vi "Routines.Compile.vi"(8 "error in (no error)":errorcluster, 11 "Section Ref in":T5 format="%.0x") -> (0 "error out":errorcluster, 1 "Routines":T1 {"Stop.Resp"."Signals"."Byte Order" items=["Little Endian", "Big Endian"]; "Stop.Resp"."Signals"."Data Type" items=["Signed", "Unsigned", "IEEE Float"]; "Stop.Cmd"."Signals"."Byte Order" items=["Little Endian", "Big Endian"]; "Stop.Cmd"."Signals"."Data Type" items=["Signed", "Unsigned", "IEEE Float"]; "Request.Resp"."Signals"."Byte Order" items=["Little Endian", "Big Endian"]; "Request.Resp"."Signals"."Data Type" items=["Signed", "Unsigned", "IEEE Float"]; "Request.Cmd"."Signals"."Byte Order" items=["Little Endian", "Big Endian"]; "Request.Cmd"."Signals"."Data Type" items=["Signed", "Unsigned", "IEEE Float"]; "Start.Resp"."Signals"."Byte Order" items=["Little Endian", "Big Endian"]; "Start.Resp"."Signals"."Data Type" items=["Signed", "Unsigned", "IEEE Float"]; "Start.Cmd"."Signals"."Byte Order" items=["Little Endian", "Big Endian"]; "Start.Cmd"."Signals"."Data Type" items=["Signed", "Unsigned", "IEEE Float"]}, 2 "Routines Refs":T6 {"Stop.Resp"."Signal Refs" format="%.0x"; "Stop.Cmd"."Signal Refs" format="%.0x"; "Request.Resp"."Signal Refs" format="%.0x"; "Request.Cmd"."Signal Refs" format="%.0x"; "Start.Resp"."Signal Refs" format="%.0x"; "Start.Cmd"."Signal Refs" format="%.0x"}, 3 "Section Ref out":T5 format="%.0x")   [LabVIEW 2015, in "Diagnostics Addon System Explorer.lvlib"]
uses:
  Diagnostics Addon System Explorer.lvlib
  <vilib>/NI Veristand/Custom Device API/Custom Device Item Ref.ctl
  Types/Routines.Refs.ctl
  Types/Frame.Ref.ctl
  Types/Routines.Compile.ctl
  Shared/Types/Frame.Compile.ctl
  Shared/Types/Type.ctl
  Shared/Types/Signal.ctl
  Types/FG.Action.ctl
  Signal.FG.vi
  <vilib>/NI Veristand/Custom Device API/NI VeriStand - Get Custom Device Channel Data.vi
  <vilib>/NI Veristand/Custom Device API/NI VeriStand - Get Item Description.vi
  <vilib>/NI Veristand/Custom Device API/NI VeriStand - Get Item Property.vi
  <vilib>/NI Veristand/Custom Device API/Get Item Property (String).vi
  <vilib>/NI Veristand/Custom Device API/Get Item Property (Double).vi
  <vilib>/NI Veristand/Custom Device API/Get Item Property (U32).vi
  <vilib>/NI/NI VeriStand Advanced SysDef API/SysDef API/SysDef.Property.Set.vi
  <vilib>/NI/NI VeriStand Advanced SysDef API/_SubVIs/SysDef.Property.Set.String.vi
  <vilib>/NI/NI VeriStand Advanced SysDef API/_SubVIs/SysDef.Property.Set.DBL.vi
  <vilib>/NI/NI VeriStand Advanced SysDef API/_SubVIs/SysDef.Property.Set.U32.vi
  Shared/SubVIs/Constants.vi
  <vilib>/NI Veristand/Custom Device Tools/Custom Device Utility Library/NI VeriStand - Search for Item by GUID.vi
  <vilib>/NI VeriStand/Custom Device Tools/Custom Device Utility Library/Custom Device Utility Library.lvlib
  <vilib>/NI VeriStand/Custom Device API/Custom Device API.lvlib
  Shared/Diagnostics Addon Shared.lvlib
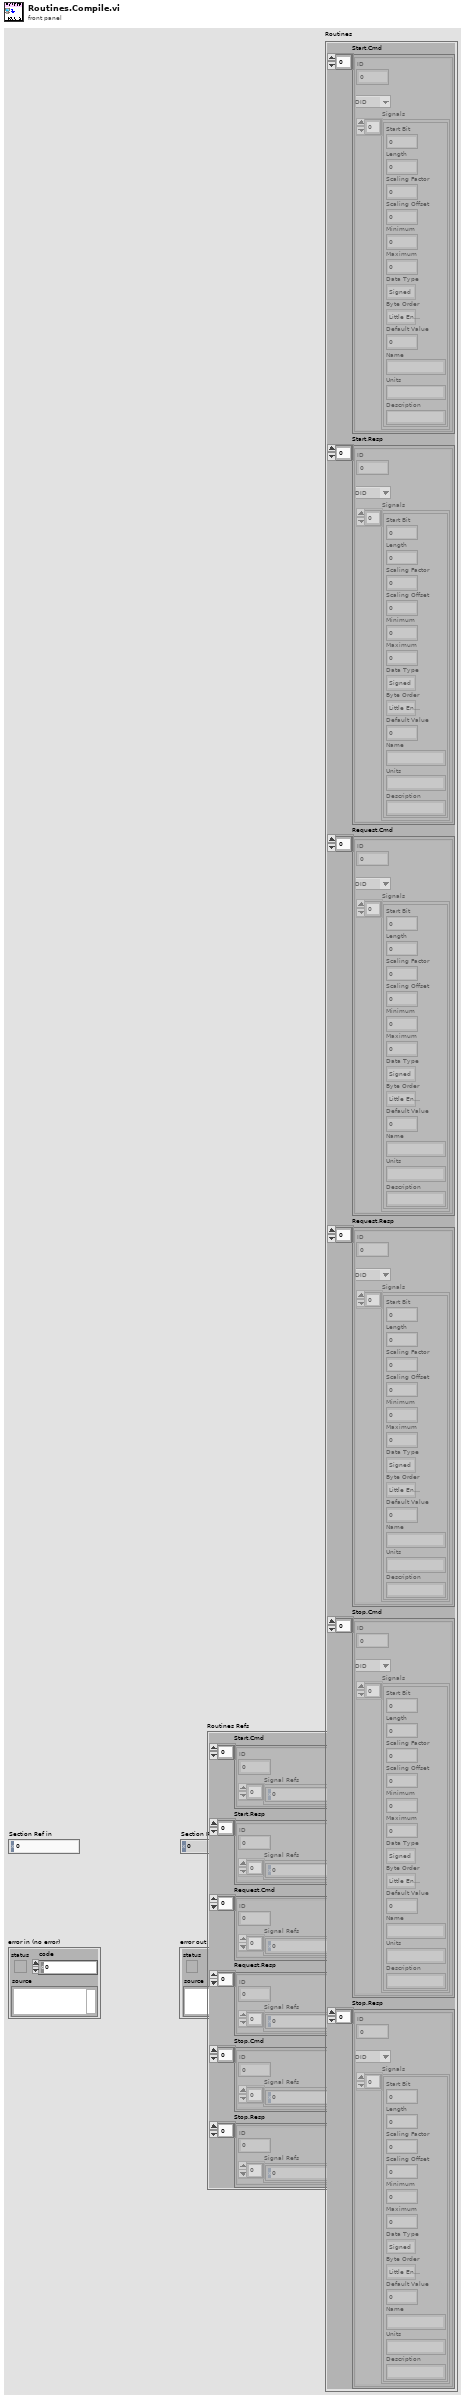
[diagram p1: front panel]
types:
  T1 = typedef "Diagnostics Addon System Explorer.lvlib/Routines.Compile.ctl" = cluster{"Start.Cmd":T2[], "Start.Resp":T2[], "Request.Cmd":T2[], "Request.Resp":T2[], "Stop.Cmd":T2[], "Stop.Resp":T2[]}
  T2 = typedef "Diagnostics Addon Shared.lvlib/Frame.Compile.ctl" = cluster{"ID":u32, "Type":T3, "Signals":T4[]}
  T3 = typedef "Diagnostics Addon Shared.lvlib/Type.ctl" = enum16{"DID", "CDID", "PID", "CPID", "Read Memory", "Write Memory", "DTC Control", "IO Cmd", "IO Resp", "Routine Start Cmd", "Routine Start Resp", "Routine Request Cmd", "Routine Request Resp", "Routine Stop Cmd", "Routine Stop Resp", "UserDefined Cmd", "UserDefined Rsp"}
  T4 = typedef "Diagnostics Addon Shared.lvlib/Signal.ctl" = cluster{"Start Bit":u32, "Length":u32, "Scaling Factor":dbl, "Scaling Offset":dbl, "Minimum":dbl, "Maximum":dbl, "Data Type":u32, "Byte Order":u32, "Default Value":dbl, "Name":string, "Units":string, "Description":string}
  T5 = typedef "Custom Device API.lvlib/Custom Device Item Ref.ctl" = u64
  T6 = typedef "Diagnostics Addon System Explorer.lvlib/Routines.Refs.ctl" = cluster{"Start.Cmd":T7[], "Start.Resp":T7[], "Request.Cmd":T7[], "Request.Resp":T7[], "Stop.Cmd":T7[], "Stop.Resp":T7[]}
  T7 = typedef "Diagnostics Addon System Explorer.lvlib/Frame.Ref.ctl" = cluster{"ID":u32, "Signal Refs":T5[]}
  T8 = typedef "Diagnostics Addon System Explorer.lvlib/FG.Action.ctl" = enum16{"Get", "Set"}
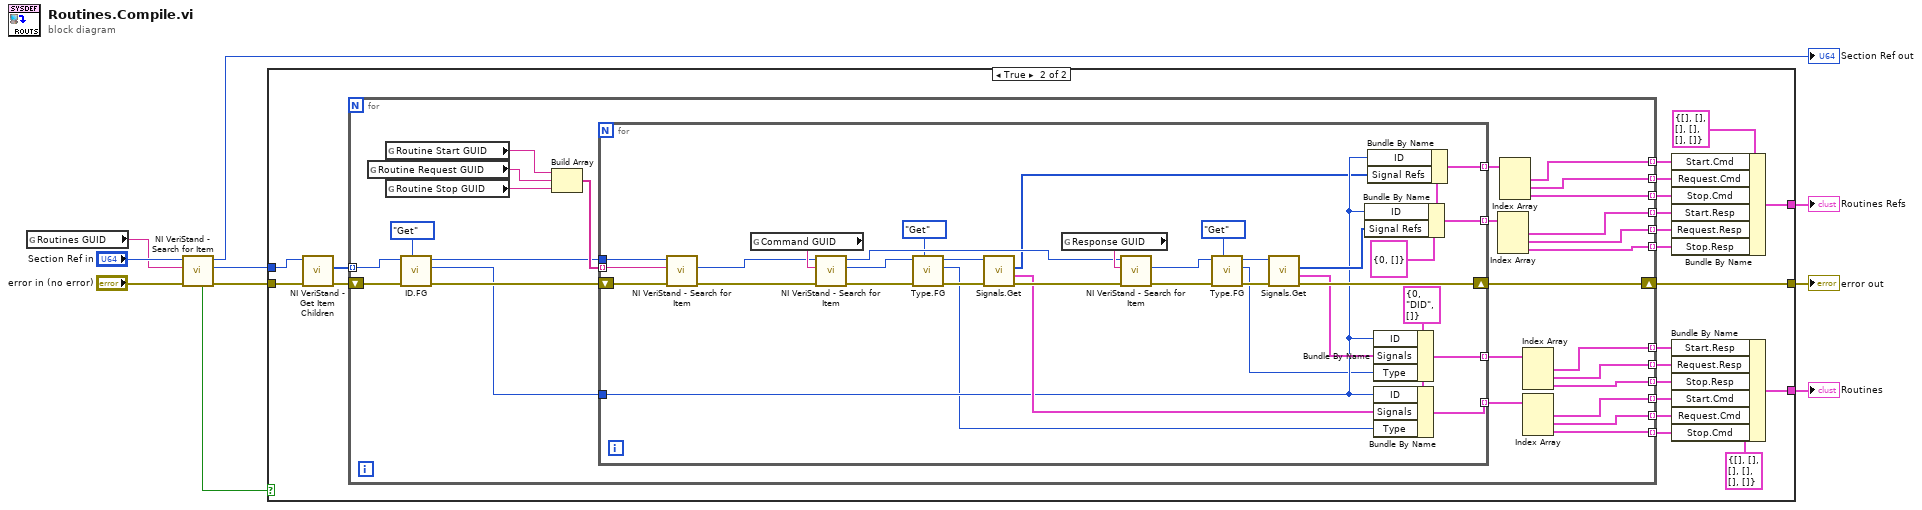
[diagram p0: block diagram]
diagram:
  n1 = global read "Constants.vi" "Routines GUID"() -> (w1:string)
  n2 = call-poly <vilib>:"NI VeriStand - Search for Item.vi"("error in"="error in (no error)", "Item GUID"=w1, "Section Ref in"="Section Ref in") -> ("error out"=w4:errorcluster, "Item Ref"=w5:T5, "Section Ref out"=→"Section Ref out":T5, "Found"=w3:bool)  [unwired: 5 in]
  n3 = case shown="True" w3 {
    tunnel: [w11 w32] -> w9
    tunnel: [_ w12] -> w8
    tunnel: w5 -> [_ w29]
    tunnel: w4 -> [w11 w28]
    tunnel: [_ w20] -> w2
    frame False {
    }
    frame True {
      n4 = call <vilib>:"NI VeriStand - Get Item Children.vi"("error in (no error)"=w28, "Item Ref in"=w29) -> ("error out"=w30:errorcluster, "Child Refs"=w31:T5[])  [unwired: 6 in, 2 out]
      n5 = for {
        shift-right: [w48] -> w32
        shift-left: w30 -> [w58]
        tunnel: w31 -> [w57] mode=indexing
        tunnel: [w46] -> w26 mode=indexing
        tunnel: [w45] -> w25 mode=indexing
        tunnel: [w44] -> w24 mode=indexing
        tunnel: [w42] -> w23 mode=indexing
        tunnel: [w41] -> w22 mode=indexing
        tunnel: [w40] -> w21 mode=indexing
        tunnel: [w38] -> w18 mode=indexing
        tunnel: [w37] -> w17 mode=indexing
        tunnel: [w36] -> w16 mode=indexing
        tunnel: [w35] -> w15 mode=indexing
        tunnel: [w34] -> w14 mode=indexing
        tunnel: [w33] -> w13 mode=indexing
        n6 = global read "Constants.vi" "Routine Request GUID"() -> (w54:string)
        n7 = global read "Constants.vi" "Routine Start GUID"() -> (w56:string)
        n8 = global read "Constants.vi" "Routine Stop GUID"() -> (w53:string)
        n9 = call "ID.FG.vi"("Action"=FG.Action."Get", "error in (no error)"=w58, "Device Item Ref in"=w57) -> ("error out"=w51:errorcluster, "ID"=w50:u32, "Device Item Ref out"=w52:T5)  [unwired: 6 in]
        n10 = Build Array(w56, w54, w53) -> (w55:string[])
        n11 = for {
          tunnel: w55 -> [w92] mode=indexing
          tunnel: w52 -> [w85]
          shift-right: [w83] -> w48
          shift-left: w51 -> [w84]
          tunnel: w50 -> [w75]
          tunnel: [w79] -> w47 mode=indexing
          tunnel: [w78] -> w43 mode=indexing
          tunnel: [w76] -> w49 mode=indexing
          tunnel: [w72] -> w39 mode=indexing
          w73 = T7 {"ID"=0, "Signal Refs"=[]} ("Status.Cmd")
          w82 = T2 {"ID"=0, "Type"=enum."DID", "Signals"=[]} ("PID In")
          n12 = call-poly <vilib>:"NI VeriStand - Search for Item.vi"("error in"=w84, "Item GUID"=w92, "Section Ref in"=w85) -> ("error out"=w86:errorcluster, "Item Ref"=w87:T5)  [unwired: 5 in, 2 out]
          n13 = global read "Constants.vi" "Command GUID"() -> (w91:string)
          n14 = call-poly <vilib>:"NI VeriStand - Search for Item.vi"("error in"=w86, "Item GUID"=w91, "Section Ref in"=w87) -> ("error out"=w70:errorcluster, "Item Ref"=w68:T5, "Section Ref out"=w89:T5)  [unwired: 5 in, 1 out]
          n15 = call "Type.FG.vi"("Action"=FG.Action."Get", "error in (no error)"=w70, "Device Item Ref in"=w68) -> ("error out"=w69:errorcluster, "Type"=w60:T3, "Device Item Ref out"=w67:T5)  [unwired: 6 in]
          n16 = call "Signals.Get.vi"("error in (no error)"=w69, "Device Item Ref out"=w67) -> ("error out"=w88:errorcluster, "Parameters"=w81:T4[], "Child Refs"=w74:T5[])  [unwired: 6 in, 1 out]
          n17 = global read "Constants.vi" "Response GUID"() -> (w90:string)
          n18 = call-poly <vilib>:"NI VeriStand - Search for Item.vi"("error in"=w88, "Item GUID"=w90, "Section Ref in"=w89) -> ("error out"=w65:errorcluster, "Item Ref"=w63:T5)  [unwired: 5 in, 2 out]
          n19 = call "Type.FG.vi"("Action"=FG.Action."Get", "error in (no error)"=w65, "Device Item Ref in"=w63) -> ("error out"=w64:errorcluster, "Type"=w61:T3, "Device Item Ref out"=w62:T5)  [unwired: 6 in]
          n20 = call "Signals.Get.vi"("error in (no error)"=w64, "Device Item Ref out"=w62) -> ("error out"=w83:errorcluster, "Parameters"=w80:T4[], "Child Refs"=w77:T5[])  [unwired: 6 in, 1 out]
          n21 = Bundle By Name(cluster=w73, "ID"=w75, "Signal Refs"=w77) -> (w76:T7)
          n22 = Bundle By Name(cluster=w73, "ID"=w75, "Signal Refs"=w74) -> (w72:T7)
          n23 = Bundle By Name(cluster=w82, "ID"=w75, "Signals"=w80, "Type"=w61) -> (w79:T2)
          n24 = Bundle By Name(cluster=w82, "ID"=w75, "Signals"=w81, "Type"=w60) -> (w78:T2)
        }
        n25 = Index Array(array=w49) -> (element #1=w35:T7, element #2=w34:T7, element #3=w33:T7)  [unwired: 3 in]
        n26 = Index Array(array=w39) -> (element #1=w38:T7, element #2=w37:T7, element #3=w36:T7)  [unwired: 3 in]
        n27 = Index Array(array=w47) -> (element #1=w46:T2, element #2=w45:T2, element #3=w44:T2)  [unwired: 3 in]
        n28 = Index Array(array=w43) -> (element #1=w42:T2, element #2=w41:T2, element #3=w40:T2)  [unwired: 3 in]
      }
      n29 = Bundle By Name(cluster=T6 {"Start.Cmd"=[], "Start.Resp"=[], "Request.Cmd"=[], "Request.Resp"=[], "Stop.Cmd"=[], "Stop.Resp"=[]} ("DIDPID Signal VS Refs"), "Start.Cmd"=w18, "Request.Cmd"=w17, "Stop.Cmd"=w16, "Start.Resp"=w15, "Request.Resp"=w14, "Stop.Resp"=w13) -> (w12:T6)
      n30 = Bundle By Name(cluster=T1 {"Start.Cmd"=[], "Start.Resp"=[], "Request.Cmd"=[], "Request.Resp"=[], "Stop.Cmd"=[], "Stop.Resp"=[]} ("Routines"), "Start.Resp"=w26, "Request.Resp"=w25, "Stop.Resp"=w24, "Start.Cmd"=w23, "Request.Cmd"=w22, "Stop.Cmd"=w21) -> (w20:T1)
    }
  }
  "error out" <- w9
  "Routines Refs" <- w8
  "Routines" <- w2
